vi "SendPoints.vi"(8 "error in (no error)":errorcluster, 9 "max points to send":i32=1000, 10 "queue in":T2, 11 "client handle":T1) -> (0 "error out":errorcluster, 1 "response":string, 2 "queue out":T2, 3 "client handle out":T1)   [LabVIEW 2022 SP3]
uses:
  <vilib>/httpClient/ClientHandle.ctl
  853a4561-62bb-48bc-97ad-d5f910773efe.vi
  <vilib>/httpClient/POSTBuffer.vi
  <vilib>/Comparison/Less/Less Functor/Less Functor.lvclass
  <vilib>/httpClient/LabVIEWHTTPClient.lvlib
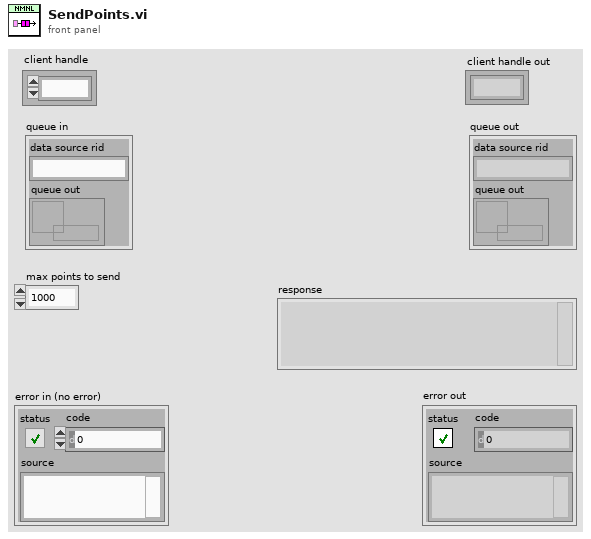
[diagram p1: front panel]
types:
  T1 = typedef "LabVIEWHTTPClient.lvlib/ClientHandle.ctl" = refnum<k1>
  T2 = cluster{"data source rid":string, "queue out":refnum<queue>}
  T3 = cluster{"channel":string, "time_seconds":i32, "time_nanos":i32, "value":dbl}
  T4 = cluster{"batches":cluster{"channel":string, "points":cluster{"type":string, "double":cluster{"timestamp":cluster{"nanos":i32, "seconds":i32}, "value":dbl}[]}}[], "dataSourceRid":string}
  T5 = cluster{"channel":string, "points":cluster{"type":string, "double":cluster{"timestamp":cluster{"nanos":i32, "seconds":i32}, "value":dbl}[]}}
  T6 = cluster{"channel":string, "time_seconds":i32, "time_nanos":i32, "value":dbl}[]
  T7 = cluster{"channel":bool, "time_seconds":bool, "time_nanos":bool, "value":bool}
  T8 = cluster{"channel":string, "points":cluster{"type":string, "double":cluster{"timestamp":cluster{"nanos":i32, "seconds":i32}, "value":dbl}[]}}[]
  T9 = cluster{"timestamp":cluster{"nanos":i32, "seconds":i32}, "value":dbl}
  T10 = cluster{"type":string, "double":cluster{"timestamp":cluster{"nanos":i32, "seconds":i32}, "value":dbl}[]}
  T11 = cluster{"timestamp":cluster{"nanos":i32, "seconds":i32}, "value":dbl}[]
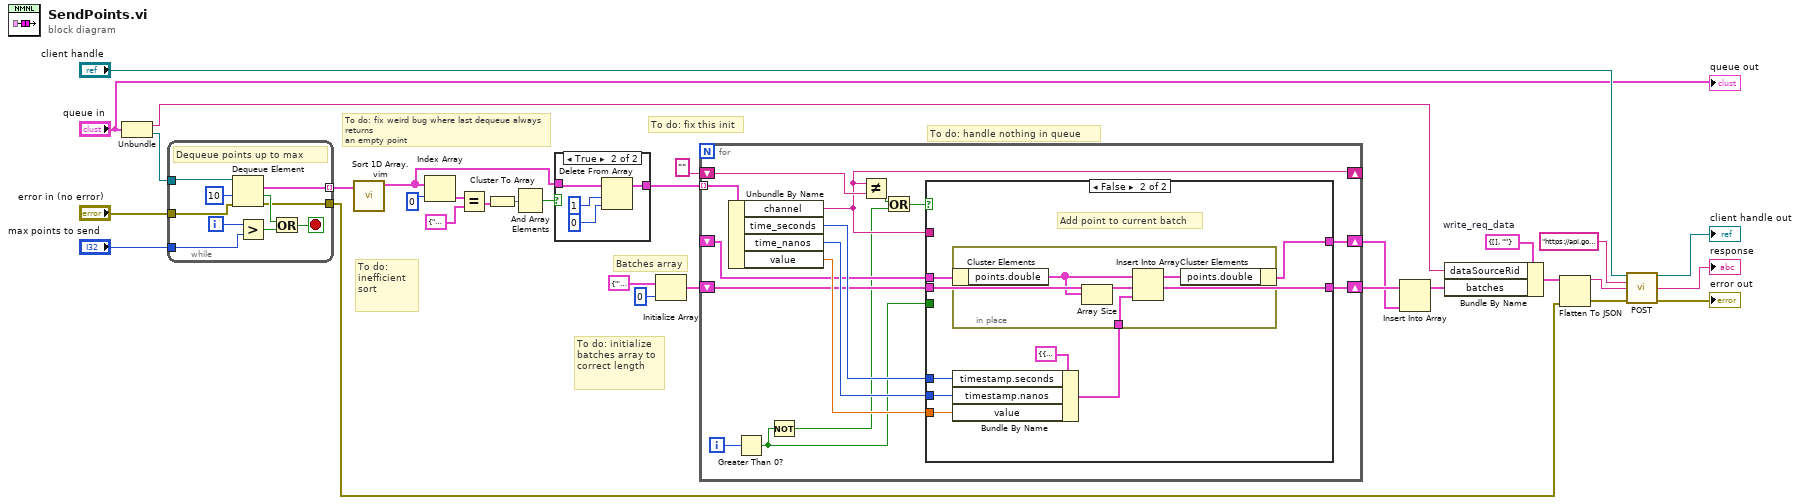
[diagram p0: block diagram]
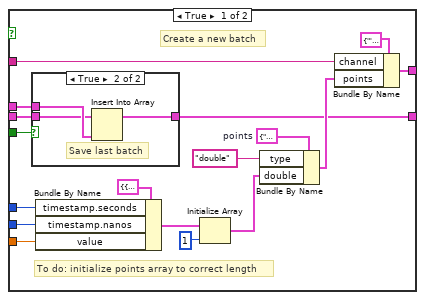
[diagram p3: hidden frame]
diagram:
  w27 = T4 {"batches"=[], "dataSourceRid"=""}  # write_req_data
  # "To do: fix weird bug where last dequeue always returns\nan empty point"
  # "To do: handle nothing in queue"
  # "To do: inefficient sort"
  # "Batches array"
  # "To do: initialize batches array to correct length"
  # "To do: fix this init"
  n1 = Unbundle("queue in") -> ("data source rid"=w2:string, "queue out"=w3:refnum<queue>)
  n2 = while {
    tunnel: w3 -> [w40]
    tunnel: [w35] -> w31 mode=indexing
    tunnel: "max points to send" -> [w34]
    tunnel: "error in (no error)" -> [w33]
    tunnel: [w32] -> w8
    i -> [w39]
    stop <- w36 stop-if-true
    # "Dequeue points up to max"
    n3 = Dequeue Element(queue=w40, timeout in ms (-1)=10, error in (no error)=w33) -> (element=w35:T3, timed out?=w38:bool, error out=w32:errorcluster)  [unwired: 1 out]
    n4 = Greater?(x=w39, y=w34) -> (0:w37:bool)
    n5 = Or(x=w38, y=w37) -> (x .or. y?=w36:bool)
  }
  n6 = call "Sort 1D Array.vim"("unsorted array"=w31) -> ("sorted array"=w14:T6)  [unwired: 10 in]
  n7 = Index Array(array=w14, index=0) -> (element=w19:T3)
  n8 = Equal?(x=w19, y=T3 {"channel"="", "time_seconds"=0, "time_nanos"=0, "value"=0.0}) -> (x = y?=w23:T7)
  n9 = Cluster To Array(cluster=w23) -> (array=w22:bool[])
  n10 = And Array Elements(Boolean array=w22) -> (logical AND=w21:bool)
  n11 = case shown="True" w21 {
    tunnel: w14 -> [w42 w45]
    tunnel: [w42 w44] -> w20
    frame False {
    }
    frame True {
      n12 = Delete From Array(array=w45, length=1, index=0) -> (array with subset deleted=w44:T6)  [unwired: 1 out]
    }
  }
  n13 = Initialize Array(T5 {"channel"="'example'", "points"={"type"="double", "double"=[]}}, 0 ("dimension size")) -> (w28:T8)
  n14 = for {
    tunnel: w20 -> [w60] mode=indexing
    shift-right: [w59] -> _
    shift-left: "" ("channel") -> [w61]
    shift-right: [w55] -> w16
    shift-left: _ -> [w54]
    shift-right: [w52] -> w17
    shift-left: w28 -> [w51]
    i -> [w53]
    n15 = Unbundle By Name(w60) -> ("channel"=w59:string, "time_seconds"=w58:i32, "time_nanos"=w57:i32, "value"=w56:dbl)
    n16 = Greater Than 0?(x=w53) -> (x > 0?=w50:bool)
    n17 = Not(x=w50) -> (.not. x?=w49:bool)
    n18 = Not Equal?(x=w59, y=w61) -> (x != y?=w48:bool)
    n19 = Or(x=w48, y=w49) -> (x .or. y?=w47:bool)
    n20 = case shown="False" w47 {
      tunnel: w59 -> [w77 _]
      tunnel: w58 -> [w71 w86]
      tunnel: w57 -> [w70 w89]
      tunnel: w56 -> [w69 w88]
      tunnel: [w67 w83] -> w55
      tunnel: w54 -> [w63 w85]
      tunnel: w51 -> [w64 w84]
      tunnel: w50 -> [w65 _]
      tunnel: [w62 w84] -> w52
      frame True {
        w76 = T10 {"type"="double", "double"=[]}  # points
        # "To do: initialize points array to correct length"
        # "Create a new batch"
        n21 = case shown="True" w65 {
          tunnel: w64 -> [w79 w81]
          tunnel: w63 -> [_ w82]
          tunnel: [w79 w80] -> w62
          frame False {
            # "First iteration"
          }
          frame True {
            # "Save last batch"
            n22 = Insert Into Array(array=w81, new element=w82) -> (w80:T8)  [unwired: 1 in]
          }
        }
        n23 = Bundle By Name(cluster=T9 {"timestamp"={"nanos"=0, "seconds"=0}, "value"=0.0}, "timestamp.seconds"=w71, "timestamp.nanos"=w70, "value"=w69) -> (w68:T9)
        n24 = Initialize Array(w68, 1 ("dimension size")) -> (w73:T11)
        n25 = Bundle By Name(cluster=w76, "type"="double", "double"=w73) -> (w66:T10)
        n26 = Bundle By Name(cluster=T5 {"channel"="'example'", "points"={"type"="double", "double"=[]}}, "channel"=w77, "points"=w66) -> (w67:T5)
      }
      frame False {
        # "Add point to current batch"
        n27 = Bundle By Name(cluster=T9 {"timestamp"={"nanos"=0, "seconds"=0}, "value"=0.0}, "timestamp.seconds"=w86, "timestamp.nanos"=w89, "value"=w88) -> (w87:T9)
        n28 = in-place {
          in-place-border: w87 -> [w94]
          n29 = in-place-cluster #1(w85) -> ("points.double"=w92:T11)
          n30 = Array Size(array=w92) -> (size(s)=w93:i32)
          n31 = Insert Into Array(array=w92, index=w93, new element=w94) -> (w91:T11)
          n32 = in-place-cluster #1("points.double"=w91) -> (w83:T5)
        }
      }
    }
  }
  n33 = Insert Into Array(array=w17, new element=w16) -> (w5:T8)  [unwired: 1 in]
  n34 = Bundle By Name(cluster=w27, "dataSourceRid"=w2, "batches"=w5) -> (w26:T4)
  n35 = Flatten To JSON(anything=w26, error in (no error)=w8) -> (JSON string=w11:string, 11:w12:errorcluster)  [unwired: 1 in]
  n36 = call-poly <vilib>:"POST.vi"("client handle"="client handle", "url"="https://api.gov.nominal.io/api/storage/writer/v1" ("Write URL"), "buffer"=w11, "error in (no error)"=w12) -> ("client handle out"=→"client handle out":T1, "body"=→"response":string, "error out"=→"error out":errorcluster)  [unwired: 8 in, 1 out]
  "queue out" <- "queue in"
